vi "MoAgSy_Engine.appendData2Variant.vi"(0 "init":variant, 2 "HGF_Agent":refnum<class "MoAgSy_AgentBase.lvclass">, 3 "kill notifier":refnum<notifier>, 5 "error in":errorcluster, 7 "VarManagerEvent":refnum<class "HGF_Event.lvclass">, 9 "HGF_Event (Monitor Event)":refnum<class "HGF_Event.lvclass">) -> (14 "dup init":variant, 19 "error out":errorcluster)   [LabVIEW 2009, in "MoAgSy.lvlib" / "MoAgSy_Engine.lvclass"]
uses:
  MoAgSy_Engine.lvclass
  MoAgSy_AgentBase/MoAgSy_AgentBase.lvclass
  HGF_BaseClasses/HGF_Event/HGF_Event.lvclass
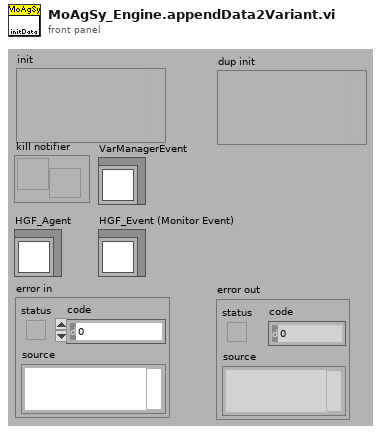
[diagram p1: front panel]
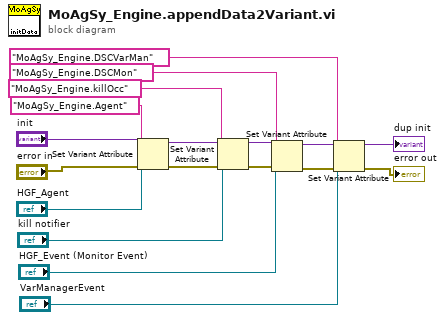
[diagram p0: block diagram]
diagram:
  n1 = Set Variant Attribute(Variant="init", name="MoAgSy_Engine.Agent", value="HGF_Agent", error in="error in") -> (Variant out=w15:variant, error out=w16:errorcluster)  [unwired: 1 out]
  n2 = Set Variant Attribute(Variant=w15, name="MoAgSy_Engine.killOcc", value="kill notifier", error in=w16) -> (Variant out=w9:variant, error out=w10:errorcluster)  [unwired: 1 out]
  n3 = Set Variant Attribute(Variant=w9, name="MoAgSy_Engine.DSCMon", value="HGF_Event (Monitor Event)", error in=w10) -> (Variant out=w7:variant, error out=w5:errorcluster)  [unwired: 1 out]
  n4 = Set Variant Attribute(Variant=w7, name="MoAgSy_Engine.DSCVarMan", value="VarManagerEvent", error in=w5) -> (Variant out=→"dup init":variant, error out=→"error out":errorcluster)  [unwired: 1 out]
